vi "Beverage_Chiller_Heater_v2.vi"() -> ()   [LabVIEW 2022 SP3]
panel:
  in  "Exit Tube Down":bool
  in  "Exit Tube Up":bool
  in  "Inlet Tube Down":bool
  in  "Inlet Tube Up":bool
  out "Water Bath Mixer On":bool
  out "Pump On":bool
  in  "Set Drink \nTemperature (F):\nCold Coffee: 33-40F\nMixed Drinks: 40-50F\nWhite Wine: 45-50F \nRed Wine: 60-68F\nBreast Milk: 99F\nHot Coffee: 120-140F":dbl=50.0
  out "Cleaning Time Remaining":i8 caption="Elapsed Time (s)"
  out "Heating":bool
  out "Cooling":bool
  in  "Water Level Sensor (On is Low)":bool
  in  "Water Temp Sensor":dbl=35.0
  in  "Drink Temp Sensor":dbl
  out "Cleaning Completed!  Remember to Drain Reservoir Before Storage":bool
  out "Drink is Ready!":bool
  out "Time to Heat or Cool":i8
  out "Drink Temp":i8
  out "Water Temp":i8
  out "Drain Reservoir and Replace with Hotter Water":bool
  out "Drain Reservoir and Replace with Ice and Water":bool
  out "Water Level Low: Add More Hot or Cold Water":bool
  in  "Start Cleaning":bool
  in  "Start Operation":bool
  in  "Mode Select":bool=TRUE
  in  "Power":bool=TRUE
  # "SETUP:\nDrain Reservoir if needed and fill with 1 qt of hot water for heating mode or 1 qt of ice+water for cooling mode. Power device on, select heating or cooling mode, and use the dial to set the desired drink temperature."
  # "OPERATION:\nAdjust positions of inlet and exit tubes into drink and when finished press \"Start Operation.\""
  # "CLEANING:\nAdjust positions of inlet tube into cleaning solution and exit tube into waste container and when finished press \"Start Cleaning.\""
  # "SENSORS:\nThese are for testing control system.  Won't be part of the user interface."
  # "OUTPUTS:\nThese are for testing control system.  Won't be part of the user interface."
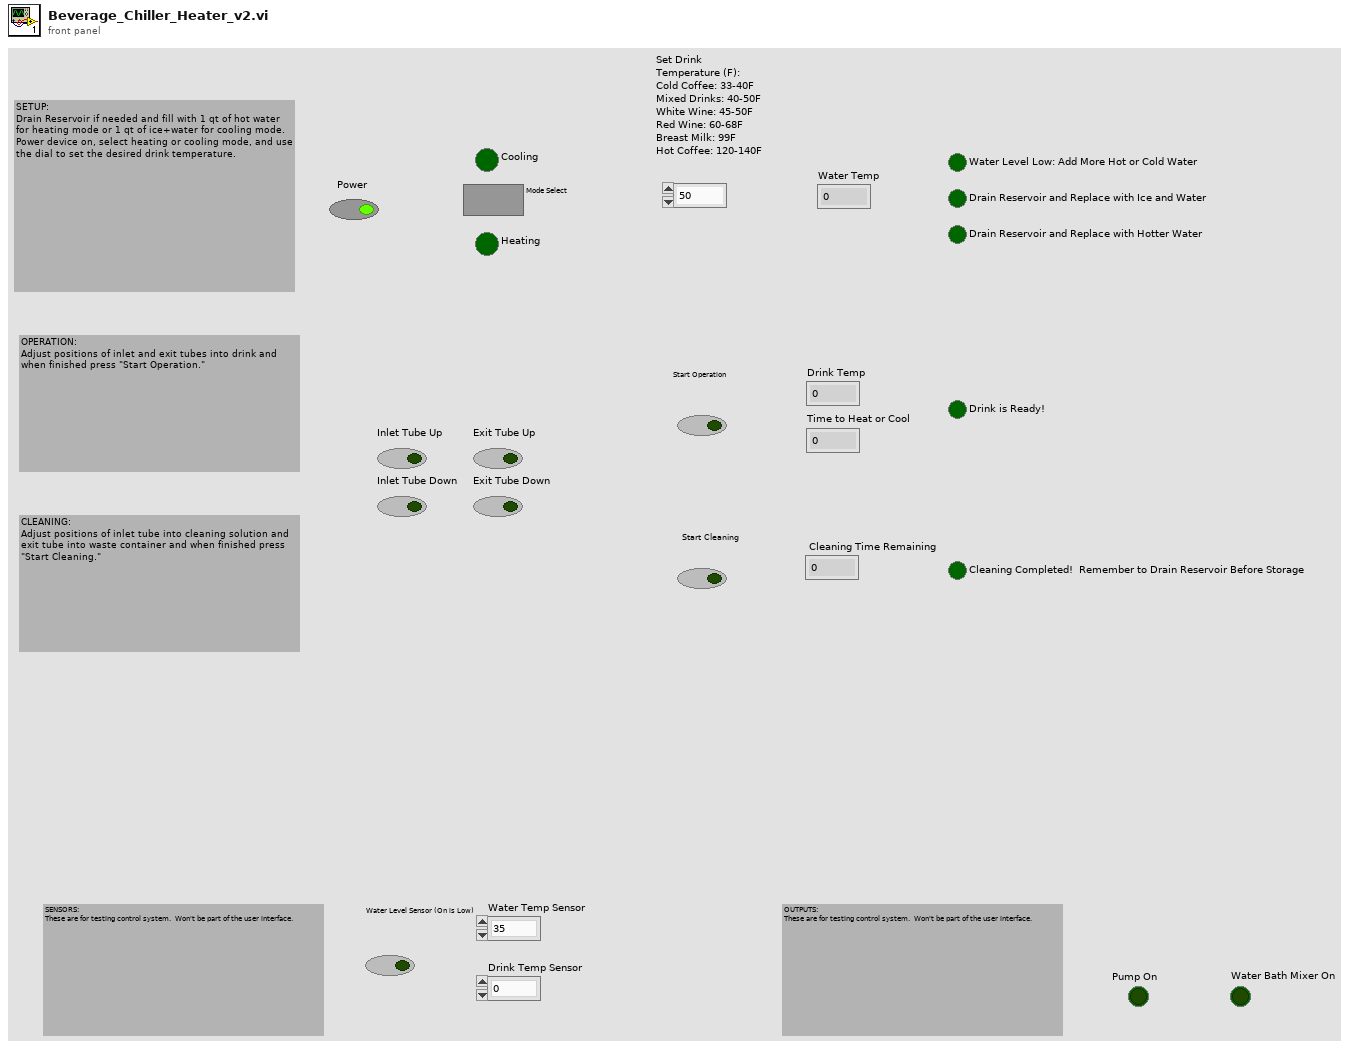
[diagram p1: front panel]
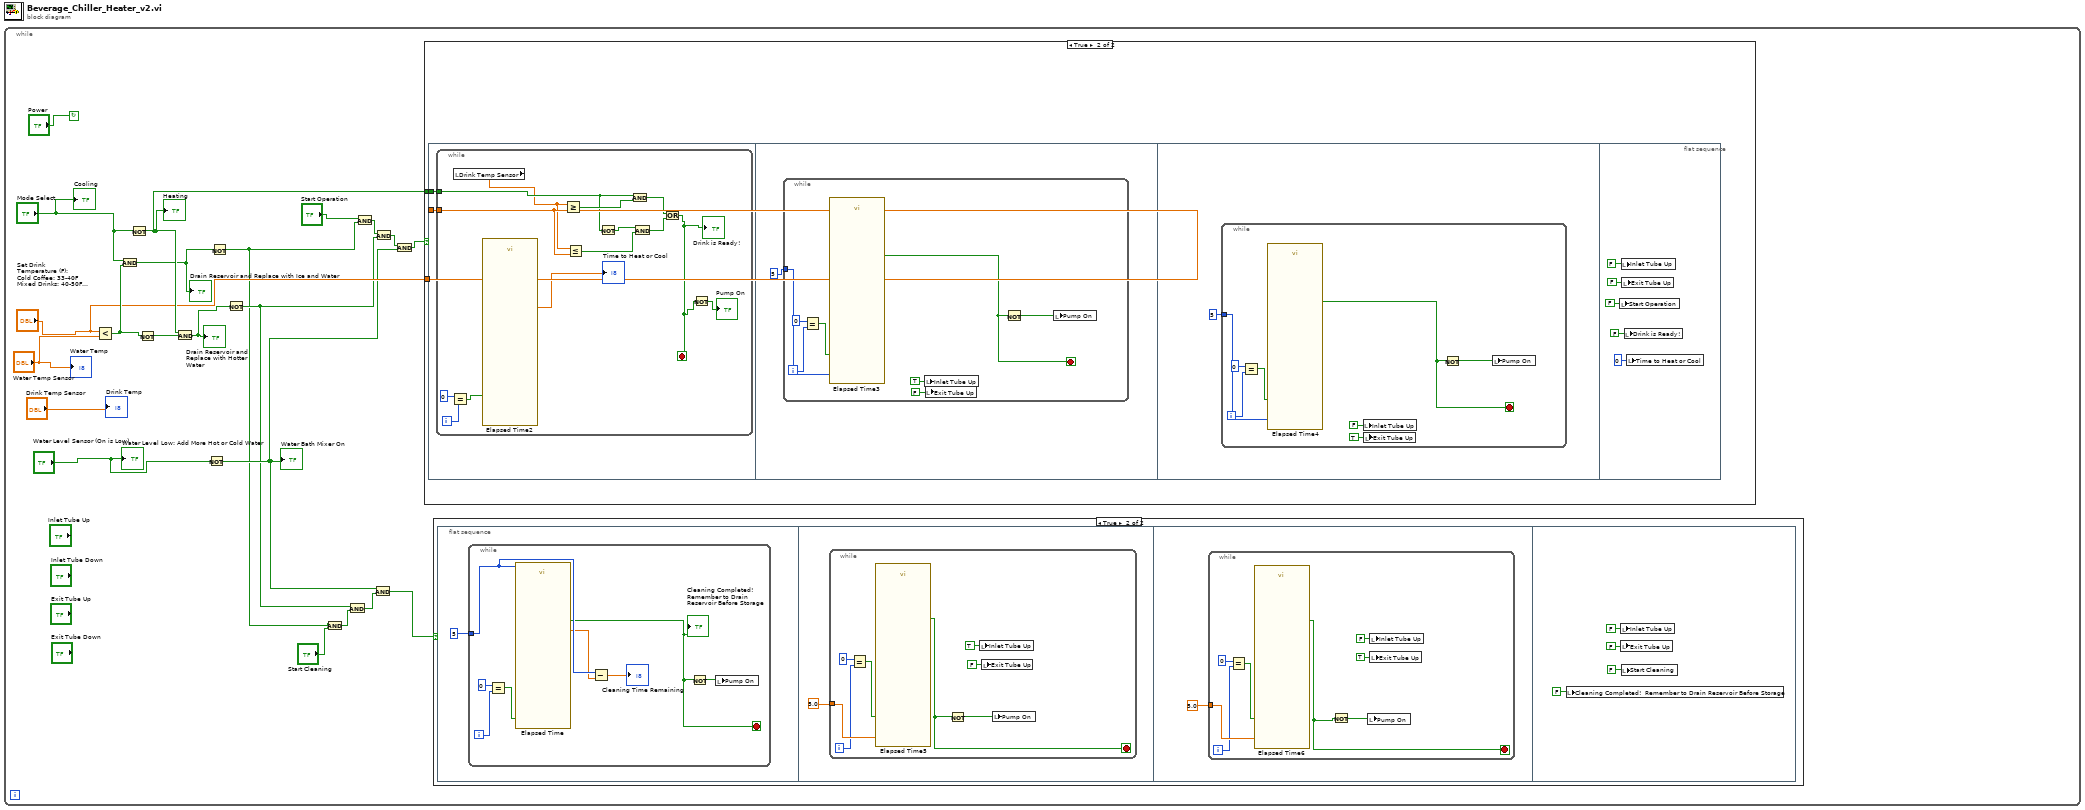
[diagram p0: block diagram]
diagram:
  n1 = while {
    stop <- "Power" continue-if-true
    n2 = Less?(x="Set Drink \nTemperature (F):\nCold Coffee: 33-40F\nMixed Drinks: 40-50F\nWhite Wine: 45-50F \nRed Wine: 60-68F\nBreast Milk: 99F\nHot Coffee: 120-140F", y="Water Temp Sensor") -> (x < y?=w22:bool)
    n3 = And(x="Mode Select", y=w22) -> (x .and. y?=w12:bool)
    "Drain Reservoir and Replace with Ice and Water" <- w12
    n4 = Not(x="Mode Select") -> (.not. x?=w18:bool)
    "Heating" <- w18
    n5 = Not(x=w22) -> (.not. x?=w21:bool)
    n6 = And(x=w18, y=w21) -> (x .and. y?=w11:bool)
    "Drain Reservoir and Replace with Hotter Water" <- w11
    n7 = Not(x="Water Level Sensor (On is Low)") -> (.not. x?=w7:bool)
    "Water Bath Mixer On" <- w7
    n8 = Not(x=w12) -> (.not. x?=w2:bool)
    n9 = Not(x=w11) -> (.not. x?=w5:bool)
    n10 = And(x=w2, y="Start Cleaning") -> (x .and. y?=w4:bool)
    n11 = And(x=w5, y=w4) -> (x .and. y?=w6:bool)
    n12 = And(x="Start Operation", y=w2) -> (x .and. y?=w10:bool)
    n13 = And(x=w7, y=w6) -> (x .and. y?=w8:bool)
    n14 = And(x=w10, y=w5) -> (x .and. y?=w9:bool)
    n15 = And(x=w9, y=w7) -> (x .and. y?=w14:bool)
    n16 = case shown="True" w14 {
      tunnel: "Set Drink \nTemperature (F):\nCold Coffee: 33-40F\nMixed Drinks: 40-50F\nWhite Wine: 45-50F \nRed Wine: 60-68F\nBreast Milk: 99F\nHot Coffee: 120-140F" -> [_ w55]
      tunnel: w18 -> [_ w54]
      frame False {
      }
      frame True {
        n17 = flat-sequence {
          tunnel: w55 -> [w57]
          tunnel: w54 -> [w56]
          frame #0 {
            n18 = while {
              tunnel: w57 -> [w64]
              tunnel: w56 -> [w66]
              i -> [w69]
              stop <- w60 stop-if-true
              n19 = Equal?(x=0, y=w69) -> (x = y?=w67:bool)
              n20 = local read "Drink Temp Sensor"() -> (w58:dbl)
              n21 = call "Elapsed Time2"("Reset"=w67) -> ("Elapsed Time (s)"=→"Time to Heat or Cool":dbl)  [unwired: 11 in, 7 out]
              n22 = Greater Or Equal?(x=w58, y=w64) -> (x >= y?=w71:bool)
              n23 = Less Or Equal?(x=w58, y=w64) -> (x <= y?=w63:bool)
              n24 = Not(x=w66) -> (.not. x?=w65:bool)
              n25 = And(x=w66, y=w71) -> (x .and. y?=w61:bool)
              n26 = And(x=w65, y=w63) -> (x .and. y?=w62:bool)
              n27 = Or(x=w61, y=w62) -> (x .or. y?=w60:bool)
              "Drink is Ready!" <- w60
              n28 = Not(x=w60) -> (.not. x?=→"Pump On":bool)
            }
          }
          frame #1 {
            n29 = while {
              tunnel: 5 -> [w77]
              i -> [w79]
              stop <- w76 stop-if-true
              n30 = Equal?(x=0, y=w79) -> (x = y?=w78:bool)
              n31 = call "Elapsed Time3"("Time Target (s)"=w77, "Reset"=w78) -> ("Time has Elapsed"=w76:bool)  [unwired: 10 in, 7 out]
              n32 = local write "Inlet Tube Up"(TRUE ("Inlet Tube Up")) -> ()
              n33 = local write "Exit Tube Up"(FALSE ("Exit Tube Up")) -> ()
              n34 = Not(x=w76) -> (.not. x?=w75:bool)
              n35 = local write "Pump On"(w75) -> ()
            }
          }
          frame #2 {
            n36 = while {
              tunnel: 5 -> [w86]
              i -> [w88]
              stop <- w85 stop-if-true
              n37 = Equal?(x=0, y=w88) -> (x = y?=w87:bool)
              n38 = call "Elapsed Time4"("Time Target (s)"=w86, "Reset"=w87) -> ("Time has Elapsed"=w85:bool)  [unwired: 10 in, 7 out]
              n39 = local write "Inlet Tube Up"(FALSE ("Inlet Tube Up")) -> ()
              n40 = local write "Exit Tube Up"(TRUE ("Exit Tube Up")) -> ()
              n41 = Not(x=w85) -> (.not. x?=w84:bool)
              n42 = local write "Pump On"(w84) -> ()
            }
          }
          frame #3 {
            n43 = local write "Start Operation"(FALSE ("Start Operation")) -> ()
            n44 = local write "Inlet Tube Up"(FALSE ("Inlet Tube Up")) -> ()
            n45 = local write "Exit Tube Up"(FALSE ("Exit Tube Up")) -> ()
            n46 = local write "Drink is Ready!"(FALSE ("Drink is Ready!")) -> ()
            n47 = local write "Time to Heat or Cool"(i8 0 ("Time to Heat or Cool")) -> ()
          }
        }
      }
    }
    n48 = case shown="True" w8 {
      frame False {
      }
      frame True {
        n49 = flat-sequence {
          frame #0 {
            n50 = while {
              tunnel: 5 -> [w28]
              i -> [w30]
              stop <- w24 stop-if-true
              n51 = Equal?(x=0, y=w30) -> (x = y?=w29:bool)
              n52 = call "Elapsed Time"("Time Target (s)"=w28, "Reset"=w29) -> ("Elapsed Time (s)"=w27:dbl, "Time has Elapsed"=w24:bool)  [unwired: 10 in, 6 out]
              "Cleaning Completed!  Remember to Drain Reservoir Before Storage" <- w24
              n53 = Subtract(x=w28, y=w27) -> (x-y=→"Cleaning Time Remaining":dbl)
              n54 = Not(x=w24) -> (.not. x?=w25:bool)
              n55 = local write "Pump On"(w25) -> ()
            }
          }
          frame #1 {
            n56 = while {
              tunnel: 5.0 ("Time Target (s)") -> [w40]
              i -> [w38]
              stop <- w36 stop-if-true
              n57 = Equal?(x=0, y=w38) -> (x = y?=w37:bool)
              n58 = call "Elapsed Time5"("Time Target (s)"=w40, "Reset"=w37) -> ("Time has Elapsed"=w36:bool)  [unwired: 10 in, 7 out]
              n59 = Not(x=w36) -> (.not. x?=w35:bool)
              n60 = local write "Inlet Tube Up"(TRUE ("Inlet Tube Up")) -> ()
              n61 = local write "Exit Tube Up"(FALSE ("Exit Tube Up")) -> ()
              n62 = local write "Pump On"(w35) -> ()
            }
          }
          frame #2 {
            n63 = while {
              tunnel: 5.0 ("Time Target (s)") -> [w49]
              i -> [w47]
              stop <- w45 stop-if-true
              n64 = Equal?(x=0, y=w47) -> (x = y?=w46:bool)
              n65 = call "Elapsed Time6"("Time Target (s)"=w49, "Reset"=w46) -> ("Time has Elapsed"=w45:bool)  [unwired: 10 in, 7 out]
              n66 = Not(x=w45) -> (.not. x?=w44:bool)
              n67 = local write "Pump On"(w44) -> ()
              n68 = local write "Inlet Tube Up"(FALSE ("Inlet Tube Up")) -> ()
              n69 = local write "Exit Tube Up"(TRUE ("Exit Tube Up")) -> ()
            }
          }
          frame #3 {
            n70 = local write "Cleaning Completed!  Remember to Drain Reservoir Before Storage"(FALSE ("Cleaning Completed!  Remember to Drain Reservoir Before Storage")) -> ()
            n71 = local write "Inlet Tube Up"(FALSE ("Inlet Tube Up")) -> ()
            n72 = local write "Exit Tube Up"(FALSE ("Exit Tube Up")) -> ()
            n73 = local write "Start Cleaning"(FALSE ("Start Cleaning")) -> ()
          }
        }
      }
    }
    "Water Temp" <- "Water Temp Sensor"
    "Water Level Low: Add More Hot or Cold Water" <- "Water Level Sensor (On is Low)"
    "Cooling" <- "Mode Select"
    "Drink Temp" <- "Drink Temp Sensor"
  }
